vi "prime number.vi"() -> ()   [LabVIEW 2020]
panel:
  out "s? t:f":string
  in  "Numeric":dbl
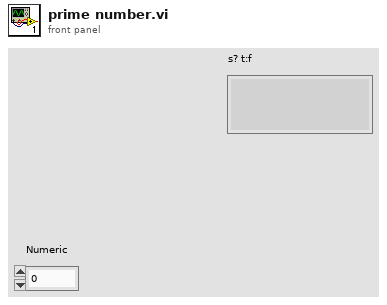
[diagram p1: front panel]
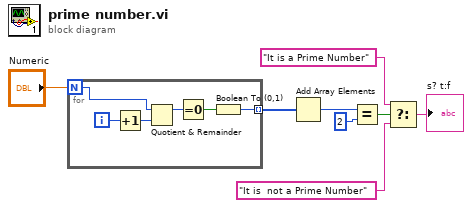
[diagram p0: block diagram]
diagram:
  n1 = for {
    N: "Numeric" -> [w12]
    tunnel: [w10] -> w7 mode=indexing
    i -> [w14]
    n2 = Increment(x=w14) -> (x+1=w13:i32)
    n3 = Quotient & Remainder(x=w12, y=w13) -> (x-y*floor(x/y)=w9:i32)  [unwired: 1 out]
    n4 = Equal To 0?(x=w9) -> (x = 0?=w11:bool)
    n5 = Boolean To (0,1)(Boolean=w11) -> (0, 1=w10:i16)
  }
  n6 = Add Array Elements(numeric array=w7) -> (sum=w6:i16)
  n7 = Equal?(x=w6, y=i16 2) -> (x = y?=w4:bool)
  n8 = Select(t="It is a Prime Number", s=w4, f="It is  not a Prime Number") -> (s? t:f=→"s? t:f":string)
